vi "spectrum_analyzer_for_testing_labview.vi"() -> ()   [LabVIEW 2023]
uses:
  <vilib>/express/express analysis/Spectral/Block/exnSpectralBlock spectral measurements PSD poly.vi
  <vilib>/express/express analysis/Spectral/Block/exnSpectralBlock spectral measurements PSD DDT.vi
  <vilib>/express/express analysis/Spectral/XNode/ExpressSpectralMeasurementsBlockNode.xnode
panel:
  out "path out":path
  in  "Save Last Trial Recording":bool
  out "Mean FF":dbl
  out "Waiting to record":bool
  out "Recording":bool
  in  "Wait to record (s)":dbl=1.0 caption="Delay Time (s)"
  out "Live Time Domain":dynamicdata(graph)
  in  "Playback Mean FF":bool
  out "# trials added":i32
  out "Stacked PSDs":dbl[][](graph)
  out "above threshold":bool=TRUE
  out "Live Fundamental Frequency":dbl
  out "Live FF PSD":dbl
  out "Live Power Spectral Density":dynamicdata(graph)
  in  "Start New Test":bool
  in  "Add Trial":bool
  in  "Trial Duration (s)":dbl=1.0 caption="Duration (s)"
  out "Mean and CI":dbl[][](graph)
  in  "stop app":bool
  # "MUST add '.wav' in name"
types:
  T1 = enum8{"Enabled", "Disabled", "Disabled and Grayed Out"}
  T2 = cluster{"averaging mode":u16, "weighting mode":u16, "number of averages":u32}
  T3 = cluster{"dB On (F)":bool, "unwrap phase (F)":bool, "convert to degree (F)":bool}
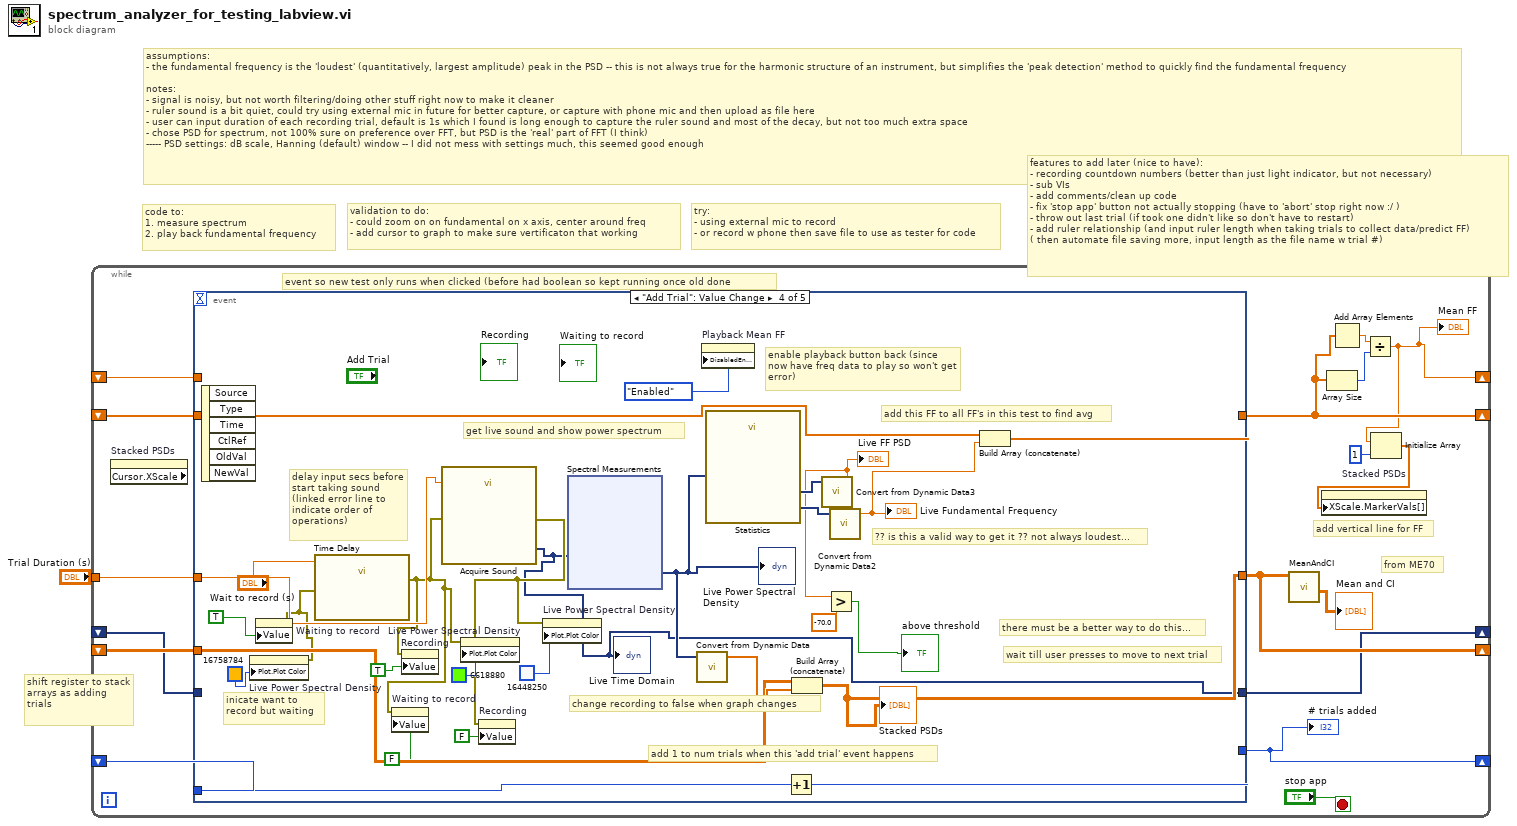
[diagram p0: block diagram]
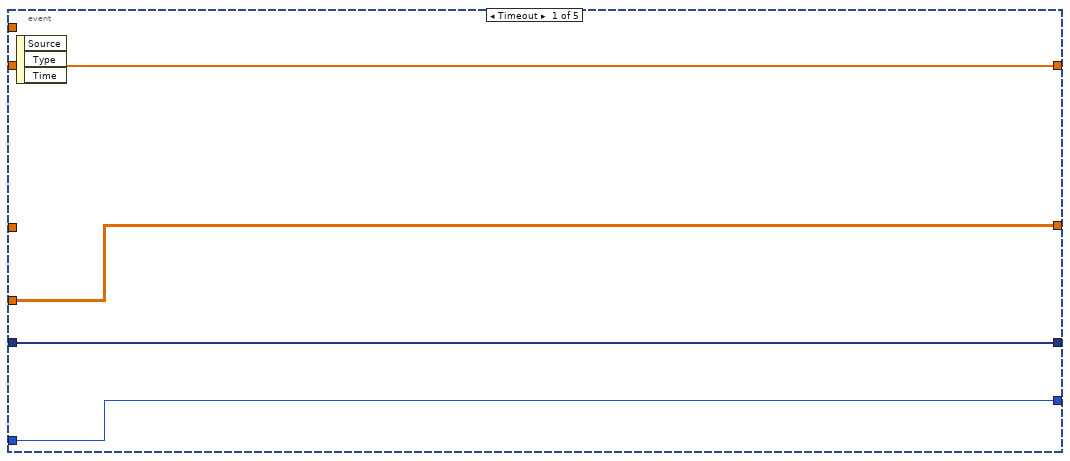
[diagram p2: hidden frame]
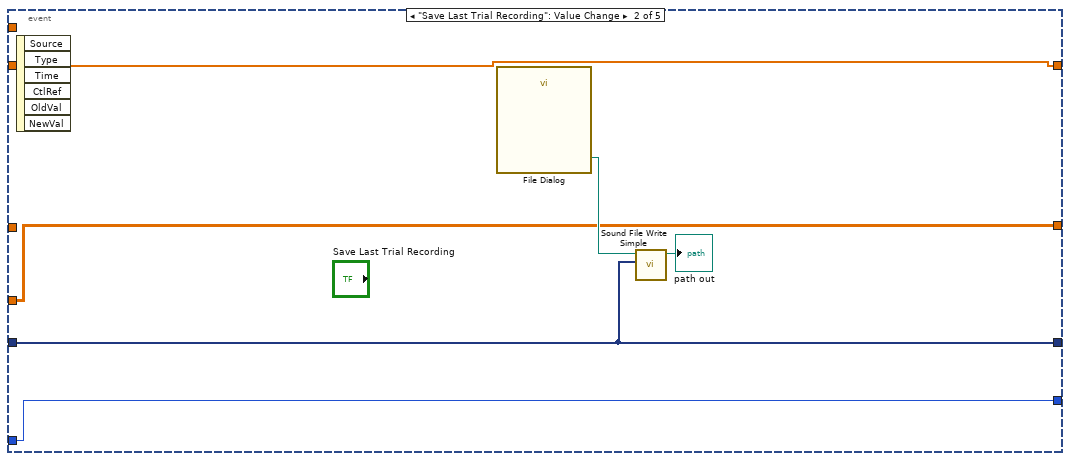
[diagram p3: hidden frame]
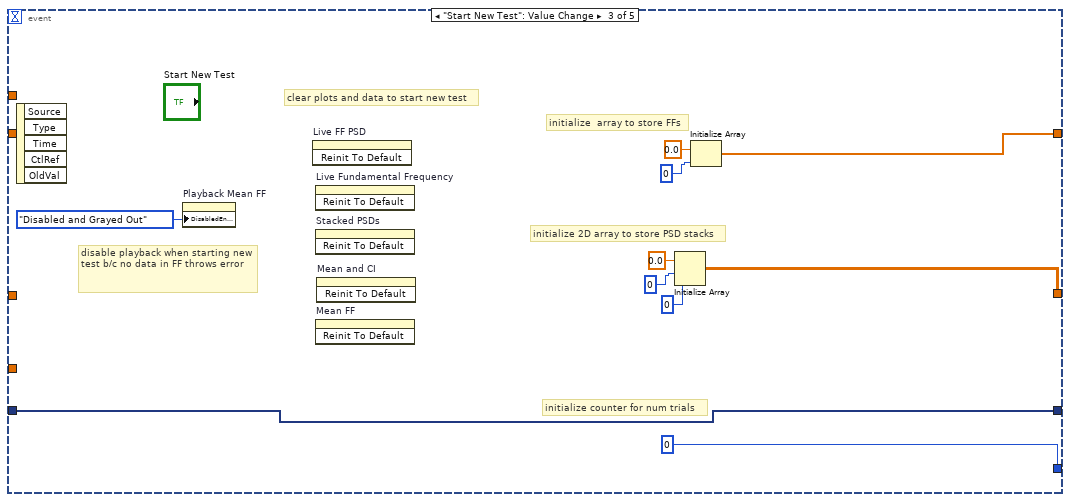
[diagram p4: hidden frame]
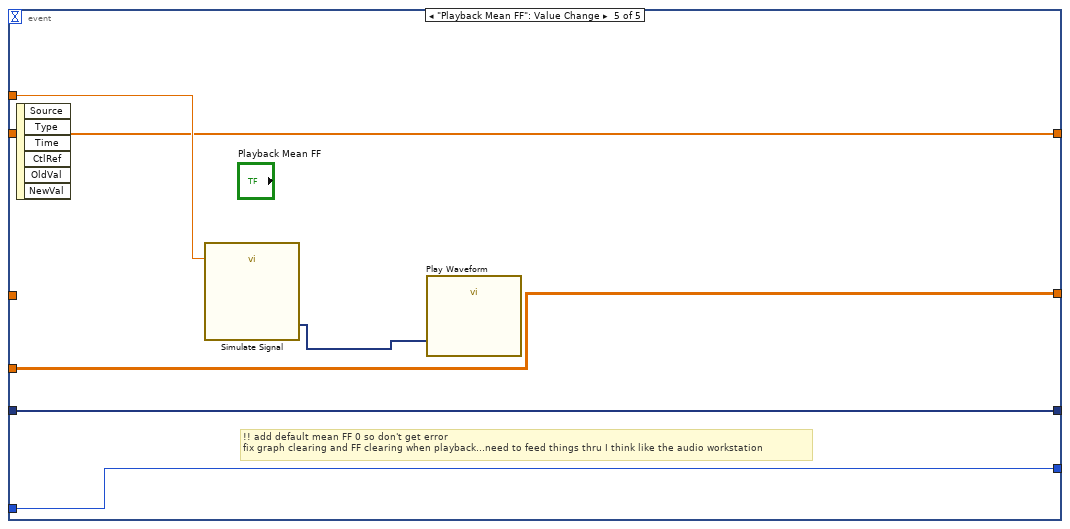
[diagram p5: hidden frame]
diagram:
  # "features to add later (nice to have):\n- recording countdown numbers (better than just light indicator, but not necessary)\n- sub VIs\n- add comments/clean up code\n- fix 'stop app' button not actually stopping (have to 'abort' stop right now :/ )\n- throw out last trial (if took one didn't like so don't have to restart)\n- add ruler relationship (and input ruler length when taking trials to collect data/predict FF)\n( then automate file saving more, input length as the file name w trial #)"
  # "shift register to stack arrays as adding trials"
  # "validation to do:\n- could zoom on on fundamental on x axis, center around freq\n- add cursor to graph to make sure vertificaton that working"
  # "assumptions:\n- the fundamental frequency is the 'loudest' (quantitatively, largest amplitude) peak in the PSD -- this is not always true for the harmonic structure of an instrument, but simplifies the 'peak detection' method to quickly find the fundamental frequency\n\nnotes:\n- signal is noisy, but not worth filtering/doing other stuff right now to make it cleaner\n- ruler sound is a bit quiet, could try using external mic in future for better capture, or capture with phone mic and then upload as file here\n- user can input duration of each recording trial, default is 1s which I found is long enough to capture the ruler sound and most of the decay, but not too much extra space\n- chose PSD for spectrum, not 100% sure on preference over FFT, but PSD is the 'real' part of FFT (I think)\n----- PSD settings: dB scale, Hanning (default) window -- I did not mess with settings much, this seemed good enough"
  # "try:\n- using external mic to record\n- or record w phone then save file to use as tester for code"
  # "code to:\n1. measure spectrum\n2. play back fundamental frequency"
  n1 = while {
    tunnel: "Trial Duration (s)" -> [w17]
    shift-right: [w14] -> _
    shift-left: _ -> [w16]
    shift-right: [w10] -> _
    shift-left: _ -> [w11]
    shift-right: [w9] -> _
    shift-left: _ -> [w8]
    shift-right: [w6] -> _
    shift-left: _ -> [w7]
    shift-right: [w3] -> _
    shift-left: _ -> [w2]
    stop <- "stop app" stop-if-true
    # "from ME70"
    # "add vertical line for FF"
    # "event so new test only runs when clicked (before had boolean so kept running once old done"
    n2 = property on="Stacked PSDs" class="WFGraph (strict)" props=["Cursor", "XScale"]() -> ()  [unwired: 2 in, 3 out]
    n3 = event shown="[3] \"Add Trial\": Value Change" {
      selector: _ -> [_ _ _ _ _]
      dyn-events: _ -> [_ _ _ _ _]
      timeout: _ -> [_ _ _ _ _]
      tunnel: w17 -> [_ _ _ w59 _]
      tunnel: w16 -> [w21 w24 _ w58 w79]
      tunnel: [w21 w24 w35 w57 w79] -> w14
      tunnel: [w22 w25 w32 w54 w78] -> w10
      tunnel: w11 -> [w22 w25 _ w56 w78]
      tunnel: [w20 w23 0 w52 w80] -> w9
      tunnel: w8 -> [w20 w23 _ w53 w80]
      tunnel: w7 -> [_ _ _ _ w81]
      tunnel: [w19 w26 w29 w39 w76] -> w3
      tunnel: w2 -> [w19 w26 w29 _ w76]
      event Timeout {
        n4 = event-data() -> ()  [unwired: 1 in, 3 out]
      }
      event "Save Last Trial Recording": Value Change {
        n5 = event-data() -> ()  [unwired: 1 in, 6 out]
        n6 = call "File Dialog"() -> ("selected path"=w28:path)  [unwired: 12 in, 3 out]
        n7 = call <vilib>:"Sound File Write Simple.vi"("data"=w26, "path"=w28) -> ("path out"=→"path out":path)  [unwired: 8 in, 1 out]
      }
      event "Start New Test": Value Change {
        # "disable playback when starting new test b/c no data in FF throws error"
        # "initialize counter for num trials"
        # "initialize  array to store FFs"
        # "initialize 2D array to store PSD stacks"
        # "clear plots and data to start new test"
        n8 = event-data() -> ()  [unwired: 1 in, 5 out]
        n9 = property on="Playback Mean FF" class="Bool"("DisabledEnum"=T1."Disabled and Grayed Out" ("Disabled")) -> ()  [unwired: 2 in, 2 out]
        n10 = invoke on="Live FF PSD" class="DigNum (strict)" method="Reinit To Default"() -> ()  [unwired: 3 in, 3 out]
        n11 = invoke on="Live Fundamental Frequency" class="DigNum (strict)" method="Reinit To Default"() -> ()  [unwired: 3 in, 3 out]
        n12 = invoke on="Stacked PSDs" class="WFGraph (strict)" method="Reinit To Default"() -> ()  [unwired: 3 in, 3 out]
        n13 = invoke on="Mean FF" class="DigNum (strict)" method="Reinit To Default"() -> ()  [unwired: 3 in, 3 out]
        n14 = invoke on="Mean and CI" class="WFGraph (strict)" method="Reinit To Default"() -> ()  [unwired: 3 in, 3 out]
        n15 = Initialize Array(0.0 ("element"), 0 ("dimension size"), 0 ("dimension size")) -> (w35:dbl[][])
        n16 = Initialize Array(0.0 ("element"), 0 ("dimension size")) -> (w32:dbl[])
      }
      event "Add Trial": Value Change {
        # "inicate want to record but waiting"
        # "enable playback button back (since now have freq data to play so won't get error)"
        # "change recording to false when graph changes"
        # "delay input secs before start taking sound (linked error line to indicate order of operations)"
        # "add 1 to num trials when this 'add trial' event happens"
        # "add this FF to all FF's in this test to find avg"
        # "get live sound and show power spectrum"
        # "wait till user presses to move to next trial"
        # "there must be a better way to do this..."
        # "?? is this a valid way to get it ?? not always loudest..."
        n17 = event-data() -> ()  [unwired: 1 in, 6 out]
        n18 = property on="Waiting to record" class="Bool (strict)"("Value"=TRUE ("Waiting to record")) -> (error out=w41:errorcluster)  [unwired: 2 in, 1 out]
        n19 = property on="Live Power Spectral Density" class="WFGraph (strict)"(error in=w41, "Plot.Plot Color"=u32 16758784) -> ()  [unwired: 1 in, 2 out]
        n20 = call "Time Delay"("error in (no error)"=w41, "Delay Time (s)"="Wait to record (s)") -> ("error out"=w45:errorcluster)  [unwired: 9 in]
        n21 = property on="Waiting to record" class="Bool (strict)"(error in=w45, "Value"=FALSE ("Waiting to record")) -> ()  [unwired: 1 in, 2 out]
        n22 = property on="Recording" class="Bool (strict)"(error in=w45, "Value"=TRUE ("Recording")) -> ()  [unwired: 1 in, 2 out]
        n23 = call "Acquire Sound"("Duration (s)"=w59, "error in (no error)"=w45) -> ("Data"=w39:dynamicdata, "error out"=w43:errorcluster)  [unwired: 16 in]
        "Live Time Domain" <- w39
        n24 = property on="Live Power Spectral Density" class="WFGraph (strict)"(error in=w45, "Plot.Plot Color"=u32 6618880) -> ()  [unwired: 1 in, 2 out]
        n25 = property on="Recording" class="Bool (strict)"(error in=w43, "Value"=FALSE ("Recording")) -> ()  [unwired: 1 in, 2 out]
        n26 = property on="Live Power Spectral Density" class="WFGraph (strict)"(error in=w43, "Plot.Plot Color"=u32 16448250) -> ()  [unwired: 1 in, 2 out]
        n27 = xnode "Spectral Measurements"("Signals"=w39) -> ("PSD"=w64:dynamicdata)  [unwired: 1 in, 1 out]
        "Live Power Spectral Density" <- w64
        n28 = call "Convert from Dynamic Data"("Dynamic Data Type"=w64) -> ("Array"=w63:dbl[])  [unwired: 3 in]
        n29 = property on="Playback Mean FF" class="Bool"("DisabledEnum"=T1."Enabled" ("Disabled")) -> ()  [unwired: 2 in, 2 out]
        n30 = call "Statistics"("Signals"=w64) -> ("Time of Maximum"=w62:dynamicdata, "Maximum"=w61:dynamicdata)  [unwired: 24 in, 1 out]
        n31 = Increment(x=w53) -> (x+1=w52:i32)
        n32 = Build Array (concatenate)(w58, w63) -> (w57:dbl[][])
        "Stacked PSDs" <- w57
        n33 = call "Convert from Dynamic Data3"("Dynamic Data Type"=w61) -> ("Scalar"=w60:dbl)  [unwired: 3 in]
        "Live FF PSD" <- w60
        n34 = Greater?(x=w60, y=-70.0 ("peak threshold")) -> (0:→"above threshold":bool)
        n35 = call "Convert from Dynamic Data2"("Dynamic Data Type"=w62) -> ("Scalar"=w55:dbl)  [unwired: 3 in]
        "Live Fundamental Frequency" <- w55
        n36 = Build Array (concatenate)(w56, w55) -> (w54:dbl[])
      }
      event "Playback Mean FF": Value Change {
        # "!! add default mean FF 0 so don't get error\nfix graph clearing and FF clearing when playback...need to feed things thru I think like the audio workstation"
        n37 = event-data() -> ()  [unwired: 1 in, 6 out]
        n38 = call "Simulate Signal"("Frequency"=w81) -> ("Sine"=w77:dynamicdata)  [unwired: 13 in, 1 out]
        n39 = call "Play Waveform"("Data"=w77) -> ()  [unwired: 18 in, 1 out]
      }
    }
    "# trials added" <- w9
    n40 = call "MeanAndCI.vi"("Array in"=w14) -> ("Mean and CI"=→"Mean and CI":dbl[][])  [unwired: 10 in]
    n41 = Array Size(array=w10) -> (size(s)=w13:i32)
    n42 = Add Array Elements(numeric array=w10) -> (sum=w12:dbl)
    n43 = Divide(x=w12, y=w13) -> (x/y=w6:dbl)
    "Mean FF" <- w6
    n44 = Initialize Array(w6, 1 ("dimension size")) -> (w4:dbl[])
    n45 = property on="Stacked PSDs" class="WFGraph (strict)"("XScale.MarkerVals[]"=w4) -> ()  [unwired: 2 in, 2 out]
  }
